vi "GetVoltage.vi"(4 "error in":errorcluster, 5 "connection ID":refnum<k5>) -> (0 "Voltage":string, 1 "error out":errorcluster, 2 "connection ID out":refnum<k5>, 3 "Answer":bool)   [LabVIEW 2013]
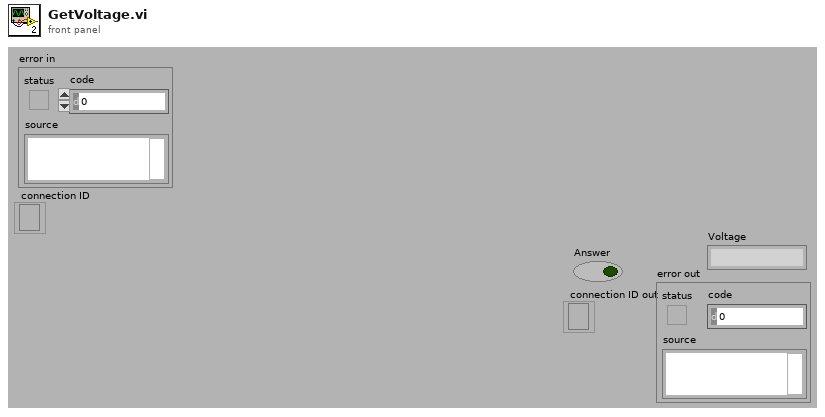
[diagram p1: front panel]
types:
  T1 = enum16{"Standard", "Buffered", "CRLF", "Immediate"}
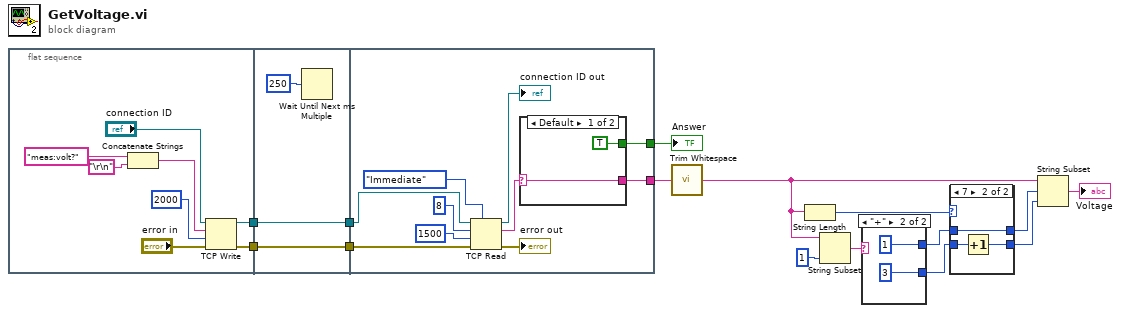
[diagram p0: block diagram]
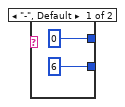
[diagram p3: hidden frame]
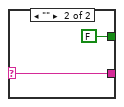
[diagram p4: hidden frame]
diagram:
  n1 = flat-sequence {
    tunnel: [w20] -> w14
    tunnel: [w19] -> w12
    tunnel: [w25] -> w15
    tunnel: w14 -> [w25]
    tunnel: [w24] -> w13
    tunnel: w12 -> [w24]
    tunnel: w15 -> [w30]
    tunnel: w13 -> [w29]
    tunnel: [w28] -> w2
    tunnel: [w27] -> w11
    frame #0 {
      n2 = Concatenate Strings("meas:volt?" ("data in"), "\r\n") -> (w17:string)
      n3 = TCP Write(connection ID="connection ID", data in=w17, error in (no error)="error in", 9:2000 ("timeout ms (25000)")) -> (connection ID out=w20:refnum<k5>, error out=w19:errorcluster)  [unwired: 1 out]
    }
    frame #1 {
      n4 = Wait Until Next ms Multiple(millisecond multiple=u32 250) -> ()  [unwired: 1 out]
    }
    frame #2 {
      n5 = TCP Read(connection ID=w30, bytes to read=8, error in (no error)=w29, 7:T1."Immediate" ("mode (standard)"), 9:1500 ("timeout ms (25000)")) -> (connection ID out=→"connection ID out":refnum<k5>, data out=w34:string, error out=→"error out":errorcluster)
      n6 = case shown="Default" w34 {
        selector: w34 -> [w38 w40]
        tunnel: [w38 w40] -> w28
        tunnel: [TRUE FALSE] -> w27
        frame Default {
        }
        frame "" {
        }
      }
    }
  }
  n7 = call <vilib>:"Trim Whitespace.vi"("string"=w2) -> ("trimmed string"=w8:string)  [unwired: 1 in]
  n8 = String Length(string=w8) -> (length=w7:i32)
  n9 = String Subset(string=w8, length (rest)=1 ("length (rest)")) -> (substring=w10:string)  [unwired: 1 in]
  n10 = case shown="\"+\"" w10 {
    tunnel: [0 ("length (rest)") 1 ("length (rest)")] -> w4
    tunnel: [6 ("length (rest)") 3 ("length (rest)")] -> w6
    frame "-", Default {
    }
    frame "+" {
    }
  }
  n11 = case shown="7" w7 {
    tunnel: w6 -> [w46 w49]
    tunnel: [w46 w48] -> w5
    tunnel: w4 -> [w45 w47]
    tunnel: [w45 w47] -> w3
    frame 6, Default {
    }
    frame 7 {
      n12 = Increment(x=w49) -> (x+1=w48:i32)
    }
  }
  n13 = String Subset(string=w8, offset (0)=w3, length (rest)=w5) -> (substring=→"Voltage":string)
  "Answer" <- w11
